vi "Data Access.vi"(8 "error in (no error)":errorcluster, 10 "Data Access Handler":refnum<class "Data Access Handler.lvclass">, 11 "Data Tracker Msg in":refnum<class "Data Tracker Msg.lvclass">) -> (0 "error out":errorcluster, 3 "Data Tracker Msg out":refnum<class "Data Tracker Msg.lvclass">)   [LabVIEW 2020, in "Data Tracker.lvlib" / "Data Tracker Msg.lvclass"]
doc: "Expose class private data to the front panel while letting the Data Access Handler class act on the data."
uses:
  Data Tracker Msg.lvclass
  C:/Current projects/WS/PPL/HDH.Actor Framework.Core.Msg.lvlibp/Flex Msg/Flex Msg.lvclass
  PPL/HDH.Actor Framework.Core.Msg.lvlibp/Flex Msg/Data Access Handlers/Data Access Handler/Data Access Handler.lvclass
  PPL/HDH.Actor Framework.Core.Actor.lvlibp/1abvi3w/vi.lib/ActorFramework/Message Enqueuer/Message Priority.ctl
  PPL/HDH.Actor Framework.Core.Publisher.lvlibp/Messages/Response Msg/Response Core/Controls/Ctl_SendFunction.ctl
  Controls/Ctl_Action.ctl
  Data Tracker Msg.lvclass/Data Tracker Msg.ctl
  PPL/HDH.Actor Framework.Core.Actor.lvlibp/1abvi3w/vi.lib/ActorFramework/Message Enqueuer/Message Enqueuer.lvclass
  PPL/HDH.Actor Framework.Core.Publisher.lvlibp
  Data Tracker.lvlib
panel:
  in  "Action":T1
  in  "Publish Data?(F)":bool
  in  "Send Function":T2
  in  "Priority":T3=enum."Normal"
  in  "Timeout if waiting":i32=-1
  in  "Cancel":bool
  in  "OK":bool
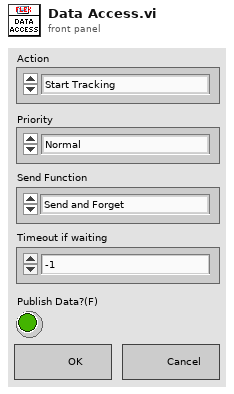
[diagram p1: front panel]
types:
  T1 = typedef "Data Tracker.lvlib/Ctl_Action.ctl" = enum16{"Start Tracking", "End Tracking", "Abort Tracking"}
  T2 = typedef "HDH.Actor Framework.Core.Publisher.lvlibp/Ctl_SendFunction.ctl" = enum16{"Send and Forget", "Request Reply", "Await Reply"}
  T3 = typedef "HDH.Actor Framework.Core.Actor.lvlibp/Message Enqueuer.lvclass/Message Priority.ctl" = enum16{"Low", "Normal", "High"}
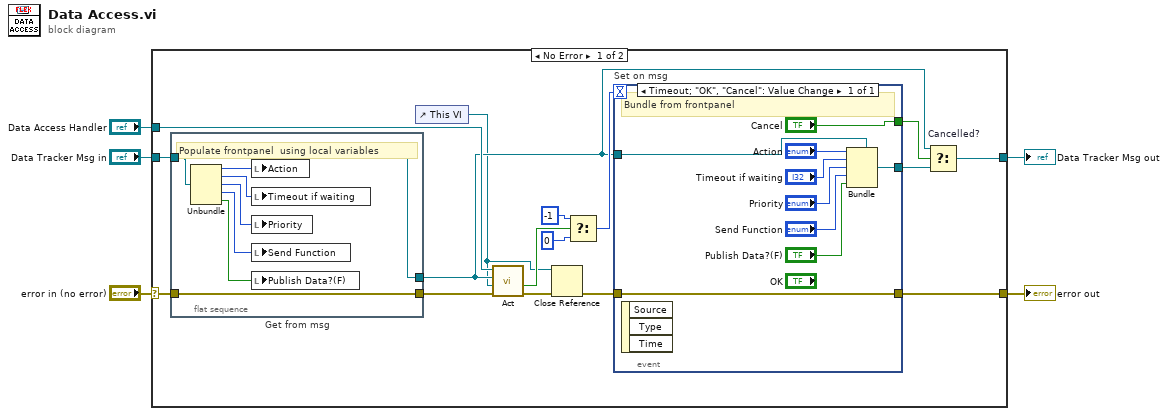
[diagram p0: block diagram]
diagram:
  n1 = case shown="No Error" "error in (no error)" {
    selector: "error in (no error)" -> [w21 w39]
    tunnel: [w14 w39] -> w4
    tunnel: [w9 w38] -> w2
    tunnel: "Data Tracker Msg in" -> [w12 w38]
    tunnel: "Data Access Handler" -> [w20 _]
    frame No Error {
      n2 = flat-sequence "Get from msg" {
        tunnel: w21 -> [w37]
        tunnel: [w36] -> w7
        tunnel: w12 -> [w36]
        tunnel: [w37] -> w19
        frame #0 {
          # "Populate frontpanel  using local variables"
          n3 = Unbundle(w36) -> (w35:T1, w34:i32, w33:T3, w32:T2, w31:bool)
          n4 = local write "Action"(w35) -> ()
          n5 = local write "Timeout if waiting"(w34) -> ()
          n6 = local write "Priority"(w33) -> ()
          n7 = local write "Send Function"(w32) -> ()
          n8 = local write "Publish Data?(F)"(w31) -> ()
        }
      }
      n9 = control-ref of="This VI"() -> (w6:refnum<vi>)
      n10 = call-dynamic "Act.vi"("error in (no error)"=w19, "VI Refnum in"=w6, "Flex Msg type"=w7, "Data Access Handler in"=w20) -> ("error out"=w11:errorcluster, "Await user action?"=w18:bool)  [unwired: 5 in, 1 out]
      n11 = Close Reference(reference=w6, error in (no error)=w11) -> (error out=w13:errorcluster)
      n12 = Select(t=-1, s=w18, f=0 ("t")) -> (s? t:f=w15:i32)
      n13 = event "Set on msg" shown="[0] Timeout;  \"OK\", \"Cancel\": Value Change" {
        selector: _ -> [_]
        dyn-events: _ -> [_]
        timeout: w15 -> [_]
        tunnel: [w30] -> w14
        tunnel: w13 -> [w30]
        tunnel: ["Cancel"] -> w10
        tunnel: [w27] -> w8
        tunnel: w7 -> [w29]
        event Timeout; "OK", "Cancel": Value Change {
          # "Bundle from frontpanel"
          n14 = event-data() -> ()  [unwired: 1 in, 3 out]
          n15 = Bundle(cluster=w29, "Action", "Timeout if waiting", "Priority", "Send Function", "Publish Data?(F)") -> (w27:refnum<class "Data Tracker Msg.lvclass">)
        }
      }
      n16 = Select "Cancelled?"(t=w7, s=w10, f=w8) -> (s? t:f=w9:refnum<class "Data Tracker Msg.lvclass">)
    }
    frame Error {
    }
  }
  "error out" <- w4
  "Data Tracker Msg out" <- w2
